vi "SafeDivide.vi"(9 "Max":dbl, 10 "y":dbl[](array[numeric]), 11 "x":dbl[](array[numeric])) -> (3 "x/y":dbl[](array[numeric]))   [LabVIEW 2013]
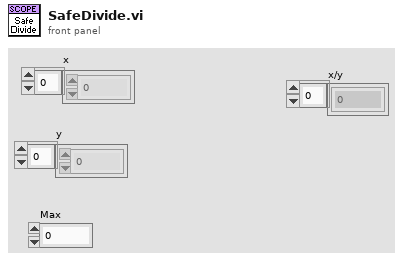
[diagram p1: front panel]
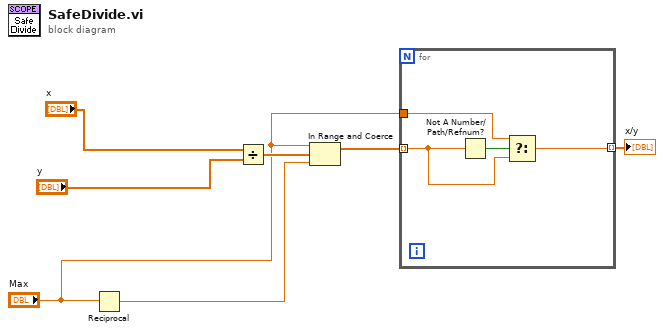
[diagram p0: block diagram]
diagram:
  n1 = Reciprocal(x="Max") -> (1/x=w4:dbl)
  n2 = Divide(x="x", y="y") -> (x/y=w7:dbl[])
  n3 = In Range and Coerce(upper limit="Max", x=w7, lower limit=w4) -> (coerced(x)=w3:dbl[])  [unwired: 1 out]
  n4 = for {
    tunnel: w3 -> [w9] mode=indexing
    tunnel: "Max" -> [w10]
    tunnel: [w8] -> w1 mode=indexing
    n5 = Not A Number/Path/Refnum?(number/path/refnum=w9) -> (NaN/Path/Refnum?=w11:bool)
    n6 = Select(t=w10, s=w11, f=w9) -> (s? t:f=w8:dbl)
  }
  "x/y" <- w1
